vi "Write applicationElements.vi"(10 "applicationElements":T1, 11 "Model in":refnum<class "Model.lvclass">) -> (3 "Model out":refnum<class "Model.lvclass">)   [LabVIEW 2013, in "Model.lvclass"]
uses:
  Model.lvclass
  ApplicationElements/ApplicationElements.ctl
  ApplicationElements/TestMonitor/TestMonitor.lvclass
  ApplicationElements/Log/TestDataLog/TestDataLog.lvclass
  ApplicationElements/FlukeDMMTC/FlukeDMMTC.lvclass
  Model.lvclass/Model.ctl
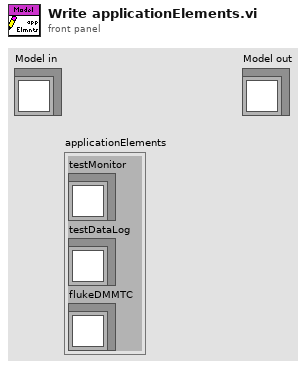
[diagram p1: front panel]
types:
  T1 = typedef "ApplicationElements.ctl" = cluster{"testMonitor":refnum<class "TestMonitor.lvclass">, "testDataLog":refnum<class "TestDataLog.lvclass">, "flukeDMMTC":refnum<class "FlukeDMMTC.lvclass">}
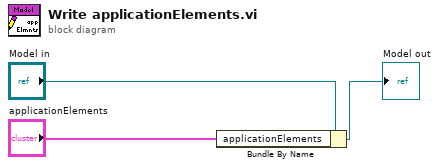
[diagram p0: block diagram]
diagram:
  n1 = Bundle By Name(cluster="Model in", "applicationElements"="applicationElements") -> (→"Model out":refnum<class "Model.lvclass">)
